vi "Open Device.vi"(8 "错误输入（无错误）":errorcluster caption="Error In(No Error)", 11 "CAN Device In":T1={"Device Type"=20, "Device Index"=0, "CANInd"=0, "Baud(E_U)"=1835016} {"Baud(E_U)" items=["1000Kbps"=393219, "800Kbps"=393220, "500Kbps"=393223, "250Kbps"=1835016, "125Kbps"=1835025, "100Kbps"=1441827, "50Kbps"=1835052, "20Kbps"=1441971, "10Kbps"=1835232, "5Kbps"=1835457]; "Device Type" items=["PCI5121"=1, "PCI9810"=2, "USBCAN1"=3, "USBCAN2"=4, "PCI9820"=5, "PCI5110"=7, "PC104CAN"=11, "CANETUDP"=12, "PCI9840B"=14, "PC104C2"=15, "PCI9820I"=16, "CANETTCP"=17, "PCIE9221"=24, "PCI5010U"=19, "USBCAN_E_U"=20, "USBCAN_2E_U"=21, "PCI5020U"=22, "PCIE9120I"=27, "PCIE9110I"=28, "PCIE9140I"=29, "USBCAN-4E-U"=31, "USBCAN-8E-U"=34]}) -> (0 "错误输出":errorcluster caption="Error Out", 1 "OPEN成功？":bool, 3 "CAN Device Out":T1={"Device Type"=20, "Device Index"=0, "CANInd"=0, "Baud(E_U)"=1835016} {"Baud(E_U)" items=["1000Kbps"=393219, "800Kbps"=393220, "500Kbps"=393223, "250Kbps"=1835016, "125Kbps"=1835025, "100Kbps"=1441827, "50Kbps"=1835052, "20Kbps"=1441971, "10Kbps"=1835232, "5Kbps"=1835457]; "Device Type" items=["PCI5121"=1, "PCI9810"=2, "USBCAN1"=3, "USBCAN2"=4, "PCI9820"=5, "PCI5110"=7, "PC104CAN"=11, "CANETUDP"=12, "PCI9840B"=14, "PC104C2"=15, "PCI9820I"=16, "CANETTCP"=17, "PCIE9221"=24, "PCI5010U"=19, "USBCAN_E_U"=20, "USBCAN_2E_U"=21, "PCI5020U"=22, "PCIE9120I"=27, "PCIE9110I"=28, "PCIE9140I"=29, "USBCAN-4E-U"=31, "USBCAN-8E-U"=34]})   [LabVIEW 2020, in "ZLGCAN.lvclass"]
uses:
  ZLGCAN.lvclass
  Device.ctl
  <vilib>/ErrorRing/Error Ring.xnode
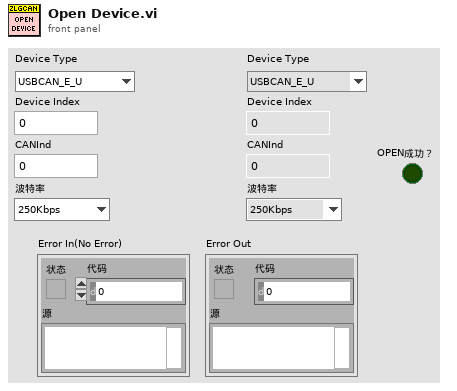
[diagram p1: front panel]
types:
  T1 = typedef "ZLGCAN.lvclass/Device.ctl" = cluster{"Device Type":u32, "Device Index":u32, "CANInd":u32, "Baud(E_U)":u32}
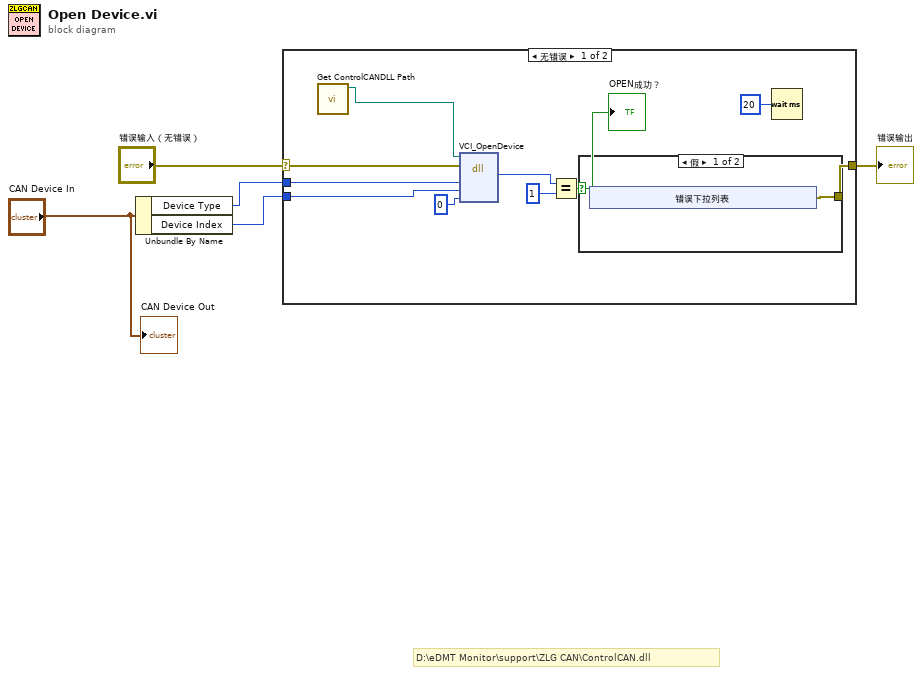
[diagram p0: block diagram]
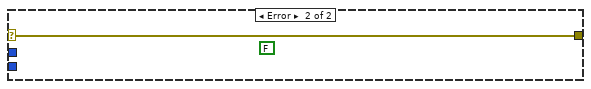
[diagram p3: hidden frame]
diagram:
  # "D:\\eDMT Monitor\\support\\ZLG CAN\\ControlCAN.dll"
  n1 = Unbundle By Name("CAN Device In") -> ("Device Type"=w4:u32, "Device Index"=w3:u32)
  n2 = case shown="无错误" "错误输入（无错误）" {
    selector: "错误输入（无错误）" -> [w12 w18]
    tunnel: [w8 w18] -> w1
    tunnel: w4 -> [w15 _]
    tunnel: w3 -> [w14 _]
    frame No Error {
      n3 = call "Get ControlCANDLL Path.vi"() -> ("拆分的路径"=w6:path)  [unwired: 10 in, 1 out]
      n4 = dll-call lib="D:/eDMT Monitor/support/ZLG CAN/ControlCAN.dll" fn="VCI_OpenDevice"(path in=w6, error in=w12, "DevType"=w15, "DevIndex"=w14, "Reserved"=u32 0) -> ("返回类型"=w7:u32)  [unwired: 4 in, 2 out]
      n5 = Equal?(x=w7, y=u32 1) -> (x = y?=w9:bool)
      "OPEN成功？" <- w9
      n6 = case shown="假" w9 {
        tunnel: [w16 _] -> w8
        frame False {
          n7 = xnode "错误下拉列表"() -> ("错误输出"=w16:errorcluster)
        }
        frame True {
        }
      }
      n8 = Wait (ms)(milliseconds to wait=u32 20 ("等待时间（毫秒）")) -> ()  [unwired: 1 out]
    }
    frame Error {
      (unwired) FALSE
    }
  }
  "错误输出" <- w1
  "CAN Device Out" <- "CAN Device In"
